vi "CAEN_HVSystem.constructor.vi"(0 "name":string, 2 "data in":string, 5 "error in(no error)":errorcluster) -> (14 "i ref out":refnum<vi>, 16 "data out":string, 19 "error out":errorcluster)   [LabVIEW 2014, in "CAEN_HVSystem.lvlib"]
doc: "This is the constructor of a class.\n\nLicense Agreement for this software:\n\nCopyright (C)\nGesellschaft für Schwerionenforschung, GSI\nPlanckstr. 1\n64291 Darmstadt\nGermany\n\nContact: D.Beck@gsi.de \n\nThis program is free software; you can redistribute it and/or modify it under the terms of the \nGNU General Public License as published by the Free Software Foundation; either version 2 of \nthe license, or (at your option) any later version.\n\nThis program is distributed in the hope that it will be useful, but WITHOUT ANY WARRANTY; \nwithout even the implied warranty of MERCHANTABILITY or FITNESS FOR A PARTICULAR PURPOSE. See the GNU General License for more details (http://www.gnu.org).\n\nGesellschaft für Schwerionenforschung, GSI\nPlanckstr. 1, 64291 Darmstadt, Germany\nFor all questions and ideas contact: M.Richter@gsi.de, H.Brand@gsi.de or D.Beck@gsi.de.\nLast update: 16-JUN-2004"
uses:
  CAEN_HVSystem.lvlib
  CAEN_HVSystem.i attribute.ctl
  CSCore/CSApplicationBaseClasses/DeviceBase/DeviceBase.myEventNames.ctl
  CSCore/CSApplicationBaseClasses/DeviceBase/DeviceBase.deviceState.ctl
  CSCore/CSApplicationBaseClasses/DeviceBase/DeviceBase.lvlib
  CSCore/CSSystem/CSSystemLib/CSSystemLib.lvlib
  CSCore/BaseProcess/BaseProcess.lvlib
  CSlibraries-extern/DimLVEvent/LVDimInterface/LVDimInterface.lvlib
panel:
  in  "CLASS.i attribute":T1 {"FrontPanOut"."FrontPanOut" format="%.0b"; "FrontPanIn"."FrontPanIn" format="%.0b"; "GenSignCfg"."GenSignCfg" format="%.0b"}
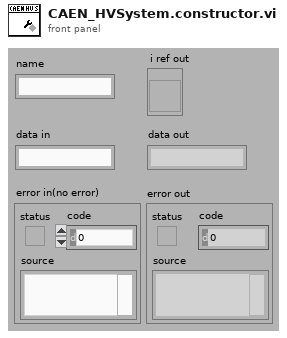
[diagram p1: front panel]
types:
  T1 = typedef "CAEN_HVSystem.lvlib/CAEN_HVSystem.i attribute.ctl" = cluster{"System Name":string, "DIM Service IDs":cluster{"Fan Status":i32}, "SymbolicName":cluster{"SymbolicName":string, "DIM Status":cluster{"no link":bool, "quality":i32, "Time Stamp":timestamp}}, "ModelName":cluster{"ModelName":string, "DIM Status":cluster{"no link":bool, "quality":i32, "Time Stamp":timestamp}}, "Slots":cluster{"Slots":i16, "DIM Status":cluster{"no link":bool, "quality":i32, "Time Stamp":timestamp}}, "Kill":cluster{"Kill":bool, "DIM Status":cluster{"no link":bool, "quality":i32, "Time Stamp":timestamp}}, "ClearAlarm":cluster{"ClearAlarm":bool, "DIM Status":cluster{"no link":bool, "quality":i32, "Time Stamp":timestamp}}, "Sessions":cluster{"Sessions":string, "DIM Status":cluster{"no link":bool, "quality":i32, "Time Stamp":timestamp}}, "SwRelease":cluster{"SwRelease":string, "DIM Status":cluster{"no link":bool, "quality":i32, "Time Stamp":timestamp}}, "GenSignCfg":cluster{"GenSignCfg":i16, "DIM Status":cluster{"no link":bool, "quality":i32, "Time Stamp":timestamp}}, "FrontPanIn":cluster{"FrontPanIn":i16, "DIM Status":cluster{"no link":bool, "quality":i32, "Time Stamp":timestamp}}, "FrontPanOut":cluster{"FrontPanOut":i16, "DIM Status":cluster{"no link":bool, "quality":i32, "Time Stamp":timestamp}}, "HvPwSM":cluster{"HvPwSM":string, "DIM Status":cluster{"no link":bool, "quality":i32, "Time Stamp":timestamp}}, "FanStat":cluster{"FanStat":string, "DIM Status":cluster{"no link":bool, "quality":i32, "Time Stamp":timestamp}}, "ClkFreq":cluster{"ClkFreq":i16, "DIM Status":cluster{"no link":bool, "quality":i32, "Time Stamp":timestamp}}, "HVClkConf":cluster{"HVClkConf":string, "DIM Status":cluster{"no link":bool, "quality":i32, "Time Stamp":timestamp}}, "CnetCrNum":cluster{"CnetCrNum":i16, "DIM Status":cluster{"no link":bool, "quality":i32, "Time Stamp":timestamp}}, "IPAddr":cluster{"IPAddr":string, "DIM Status":cluster{"no link":bool, "quality":i32, "Time Stamp":timestamp}}, "IPNetMsk":cluster{"IPNetMsk":string, "DIM Status":cluster{"no link":bool, "quality":i32, "Time Stamp":timestamp}}, "IPGw":cluster{"IPGw":string, "DIM Status":cluster{"no link":bool, "quality":i32, "Time Stamp":timestamp}}, "RS232Par":cluster{"RS232Par":string, "DIM Status":cluster{"no link":bool, "quality":i32, "Time Stamp":timestamp}}}
  T2 = enum16{"SetAttribute", "GetAttribute", "CreateAttribute", "DestroyAttribute", "DestroyAllAtributes"}
  T3 = typedef "DeviceBase.lvlib/DeviceBase.deviceState.ctl" = i16
  T4 = typedef "DeviceBase.lvlib/DeviceBase.myEventNames.ctl" = enum16{"lvmsg://Initialize", "lvmsg://Close", "lvmsg://Configure", "lvmsg://Reset", "lvmsg://IDQuery"}
  T5 = typedef "BaseProcess.lvlib/BaseProcess.i attribute.ctl" = cluster{"EventStatus":string, "EventError":i32, "PresetEvtWatchD":i32, "PresetPdcWatchD":i32, "EventTimeout":i32, "PeriodicInterval":i32, "Interface":string[], "Address":string[], "Special":string[], "PeriodicError":i32, "PeriodicStatus":string, "SuperProc":string, "Descriptors":T6[], "CaseRef":refnum<vi>, "PdcRef":refnum<vi>, "Thread Ref":refnum<vi>, "eventErrorID":i32, "eventStatusID":i32, "periodicErrorID":i32, "periodicStatusID":i32, "pdcCtrID":i32}
  T6 = typedef "BaseProcess.lvlib/BaseProcess.descriptor definition.ctl" = cluster{"selector":string, "descriptor":T7}
  T7 = typedef "BaseProcess.lvlib/BaseProcess.descriptor string definition.ctl" = string
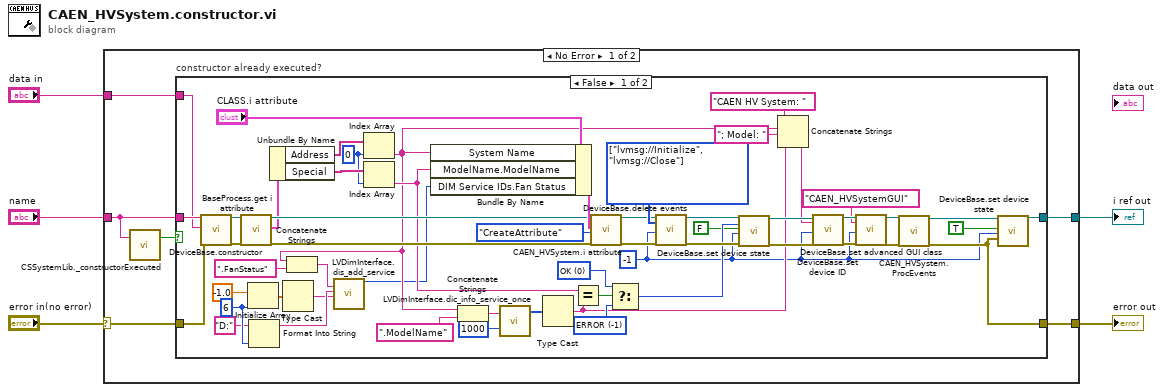
[diagram p0: block diagram]
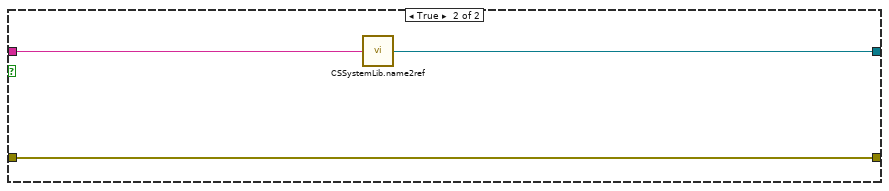
[diagram p2: hidden frame]
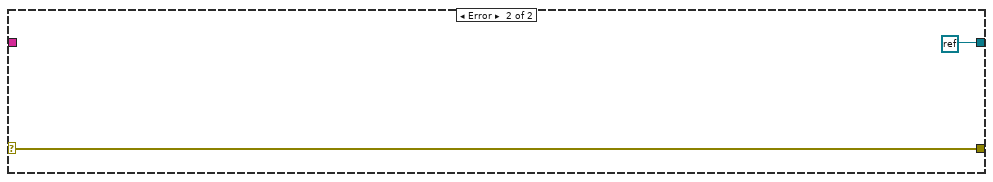
[diagram p3: hidden frame]
diagram:
  n1 = case shown="No Error" "error in(no error)" {
    selector: "error in(no error)" -> [w9 w70]
    tunnel: "name" -> [w8 _]
    tunnel: [w11 refnum<k0> refnum] -> w4
    tunnel: [w10 w70] -> w3
    tunnel: "data in" -> [w6 _]
    frame No Error {
      n2 = call "CSSystemLib._constructorExecuted.vi"("name"=w8) -> ("constructor executed?"=w7:bool)  [unwired: 18 in]
      n3 = case "constructor already executed?" shown="False" w7 {
        tunnel: w8 -> [w65 w69]
        tunnel: [w47 w68] -> w11
        tunnel: [w28 w67] -> w10
        tunnel: w9 -> [w64 w67]
        tunnel: w6 -> [w63 _]
        frame False {
          w38 = T3 -1 items=["ERROR"=-1, "OK"=0, "NOT_OK"=1] ("deviceState")
          w39 = T3 0 items=["ERROR"=-1, "OK"=0, "NOT_OK"=1] ("deviceState")
          w62 = T4[] [enum."lvmsg://Initialize", enum."lvmsg://Close"] items=["lvmsg://Initialize", "lvmsg://Close", "lvmsg://Configure", "lvmsg://Reset", "lvmsg://IDQuery"] ("events")
          w26 = 6 ("dimension size")
          w52 = 0 ("index")
          w13 = -1 ("ms timeout (10000)")
          n4 = call "DeviceBase.constructor.vi"("name"=w65, "data in"=w63, "error in (no error)"=w64) -> ("i ref out"=w58:refnum<vi>, "error out"=w59:errorcluster)  [unwired: 14 in, 1 out]
          n5 = call "BaseProcess.get i attribute.vi"("i ref in"=w58, "error in (no error)"=w59) -> ("i ref out"=w56:refnum<vi>, "i attribute"=w55:T5, "error out"=w57:errorcluster)  [unwired: 15 in]
          n6 = Initialize Array(-1.0, w26) -> (w23:dbl[])
          n7 = Format Into String(initial string="D:", w26) -> (resulting string=w24:string)  [unwired: 2 in, 1 out]
          n8 = Unbundle By Name(w55) -> ("Address"=w54:string[], "Special"=w53:string[])
          n9 = Type Cast(x=w23) -> (*(type *) &x=w22:string)  [unwired: 1 in]
          n10 = Index Array(array=w54, index=w52) -> (element=w20:string)
          n11 = Concatenate Strings(w20, ".FanStatus" ("string")) -> (w21:string)
          n12 = call "LVDimInterface.dis_add_service.vi"("serviceName"=w21, "typeDescriptor"=w24, "data"=w22) -> ("my_serviceID"=w18:i32)  [unwired: 15 in, 1 out]
          n13 = Index Array(array=w53, index=w52) -> (element=w45:string)
          n14 = Bundle By Name(cluster="CLASS.i attribute", "System Name"=w20, "ModelName.ModelName"=w45, "DIM Service IDs.Fan Status"=w18) -> (w60:T1)
          n15 = Concatenate Strings(w20, ".ModelName" ("string")) -> (w50:string)
          n16 = call "LVDimInterface.dic_info_service_once.vi"("serviceName"=w50, "timeout [ms]"=u32 1000) -> ("data"=w46:i8[])  [unwired: 14 in, 3 out]
          n17 = Type Cast(x=w46) -> (*(type *) &x=w33:string)  [unwired: 1 in]
          n18 = Equal?(x=w45, y=w33) -> (x = y?=w40:bool)
          n19 = call "CAEN_HVSystem.i attribute.vi"("VI Refnum"=w56, "CLASS.i attribute"=w60, "Action"=T2."CreateAttribute", "error in (no error)"=w57) -> ("VI Refnum out"=w31:refnum<vi>, "error out"=w30:errorcluster)  [unwired: 13 in, 1 out]
          n20 = Select(t=w39, s=w40, f=w38) -> (s? t:f=w37:T3)
          n21 = call "DeviceBase.delete events.vi"("i ref in"=w31, "events"=w62, "ms timeout (10000)"=w13, "error in (no error)"=w30) -> ("i ref out"=w43:refnum<vi>, "error out"=w44:errorcluster)  [unwired: 13 in, 1 out]
          n22 = call "DeviceBase.set device state.vi"("i ref in"=w43, "deviceState"=w37, "implicit"=FALSE, "ms timeout (10000)"=w13, "error in (no error)"=w44) -> ("i ref out"=w42:refnum<vi>, "error out"=w41:errorcluster)  [unwired: 12 in, 1 out]
          n23 = Concatenate Strings("CAEN HV System: " ("string"), w20, "; Model: " ("string"), w33) -> (w32:string)
          n24 = call "DeviceBase.set device ID.vi"("i ref in"=w42, "deviceID"=w32, "ms timeout (10000)"=w13, "error in (no error)"=w41) -> ("i ref out"=w15:refnum<vi>, "error out"=w16:errorcluster)  [unwired: 13 in, 1 out]
          n25 = call "DeviceBase.set advanced GUI class.vi"("i ref in"=w15, "advancedGUIClass"="CAEN_HVSystemGUI", "ms timeout (10000)"=w13, "error in (no error)"=w16) -> ("i ref out"=w14:refnum<vi>, "error out"=w17:errorcluster)  [unwired: 13 in, 1 out]
          n26 = call "CAEN_HVSystem.ProcEvents.vi"("i ref in"=w14, "error in"=w17) -> ("i ref out"=w29:refnum<vi>, "error out"=w28:errorcluster)  [unwired: 16 in]
          n27 = call "DeviceBase.set device state.vi"("i ref in"=w29, "implicit"=TRUE, "ms timeout (10000)"=w13, "device error"=w28) -> ("i ref out"=w47:refnum<vi>)  [unwired: 13 in, 2 out]
        }
        frame True {
          n28 = call "CSSystemLib.name2ref.vi"("name"=w69) -> ("obj refnum"=w68:refnum<vi>)
        }
      }
    }
    frame Error {
    }
  }
  "i ref out" <- w4
  "error out" <- w3
